vi "Hindbrain Main With Simulator.vi"(11 "NotifierReff":T1) -> ()   [LabVIEW 2013]
doc: "Place to hold all the hindbrain code."
uses:
  Data/TypeDefs/Notifiers.ctl
  Data/TypeDefs/UTM Location.ctl
  Data/TypeDefs/Sail Set Suggestions.ctl
  Data/TypeDefs/Rudder Set Suggestions.ctl
  Data/TypeDefs/OverrideInformation.ctl
  Data/TypeDefs/OverrideMode.ctl
  Data/TypeDefs/MotorSetup.ctl
  Data/TypeDefs/DynamixelSetupInfo.ctl
  Data/TypeDefs/AirmarStatus.ctl
  Data/TypeDefs/HardwareOnline.ctl
  Data/TypeDefs/DynamixelCycleTracker.ctl
  Data/TypeDefs/RC Input Values.ctl
  Classes/Waypoint/Waypoint.lvclass
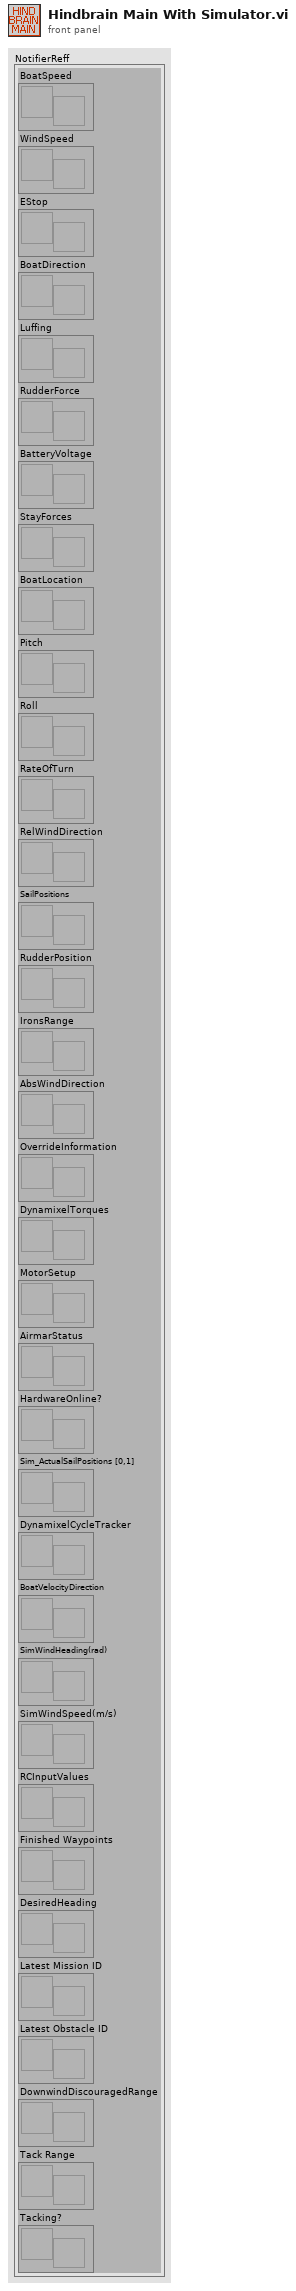
[diagram p1: front panel]
types:
  T1 = typedef "Notifiers.ctl" = cluster{"BoatSpeed":refnum<notifier>, "WindSpeed":refnum<notifier>, "EStop":refnum<notifier>, "BoatDirection":refnum<notifier>, "Luffing":refnum<notifier>, "RudderForce":refnum<notifier>, "BatteryVoltage":refnum<notifier>, "StayForces":refnum<notifier>, "BoatLocation":refnum<notifier>, "Pitch":refnum<notifier>, "Roll":refnum<notifier>, "RateOfTurn":refnum<notifier>, "RelWindDirection":refnum<notifier>, "SailPositions":refnum<notifier>, "RudderPosition":refnum<notifier>, "IronsRange":refnum<notifier>, "AbsWindDirection":refnum<notifier>, "OverrideInformation":refnum<notifier>, "DynamixelTorques":refnum<notifier>, "MotorSetup":refnum<notifier>, "AirmarStatus":refnum<notifier>, "HardwareOnline?":refnum<notifier>, "Sim_ActualSailPositions [0,1]":refnum<notifier>, "DynamixelCycleTracker":refnum<notifier>, "BoatVelocityDirection":refnum<notifier>, "SimWindHeading(rad)":refnum<notifier>, "SimWindSpeed(m/s)":refnum<notifier>, "RCInputValues":refnum<notifier>, "Finished Waypoints":refnum<notifier>, "DesiredHeading":refnum<notifier>, "Latest Mission ID":refnum<notifier>, "Latest Obstacle ID":refnum<notifier>, "DownwindDiscouragedRange":refnum<notifier>, "Tack Range":refnum<notifier>, "Tacking?":refnum<notifier>}
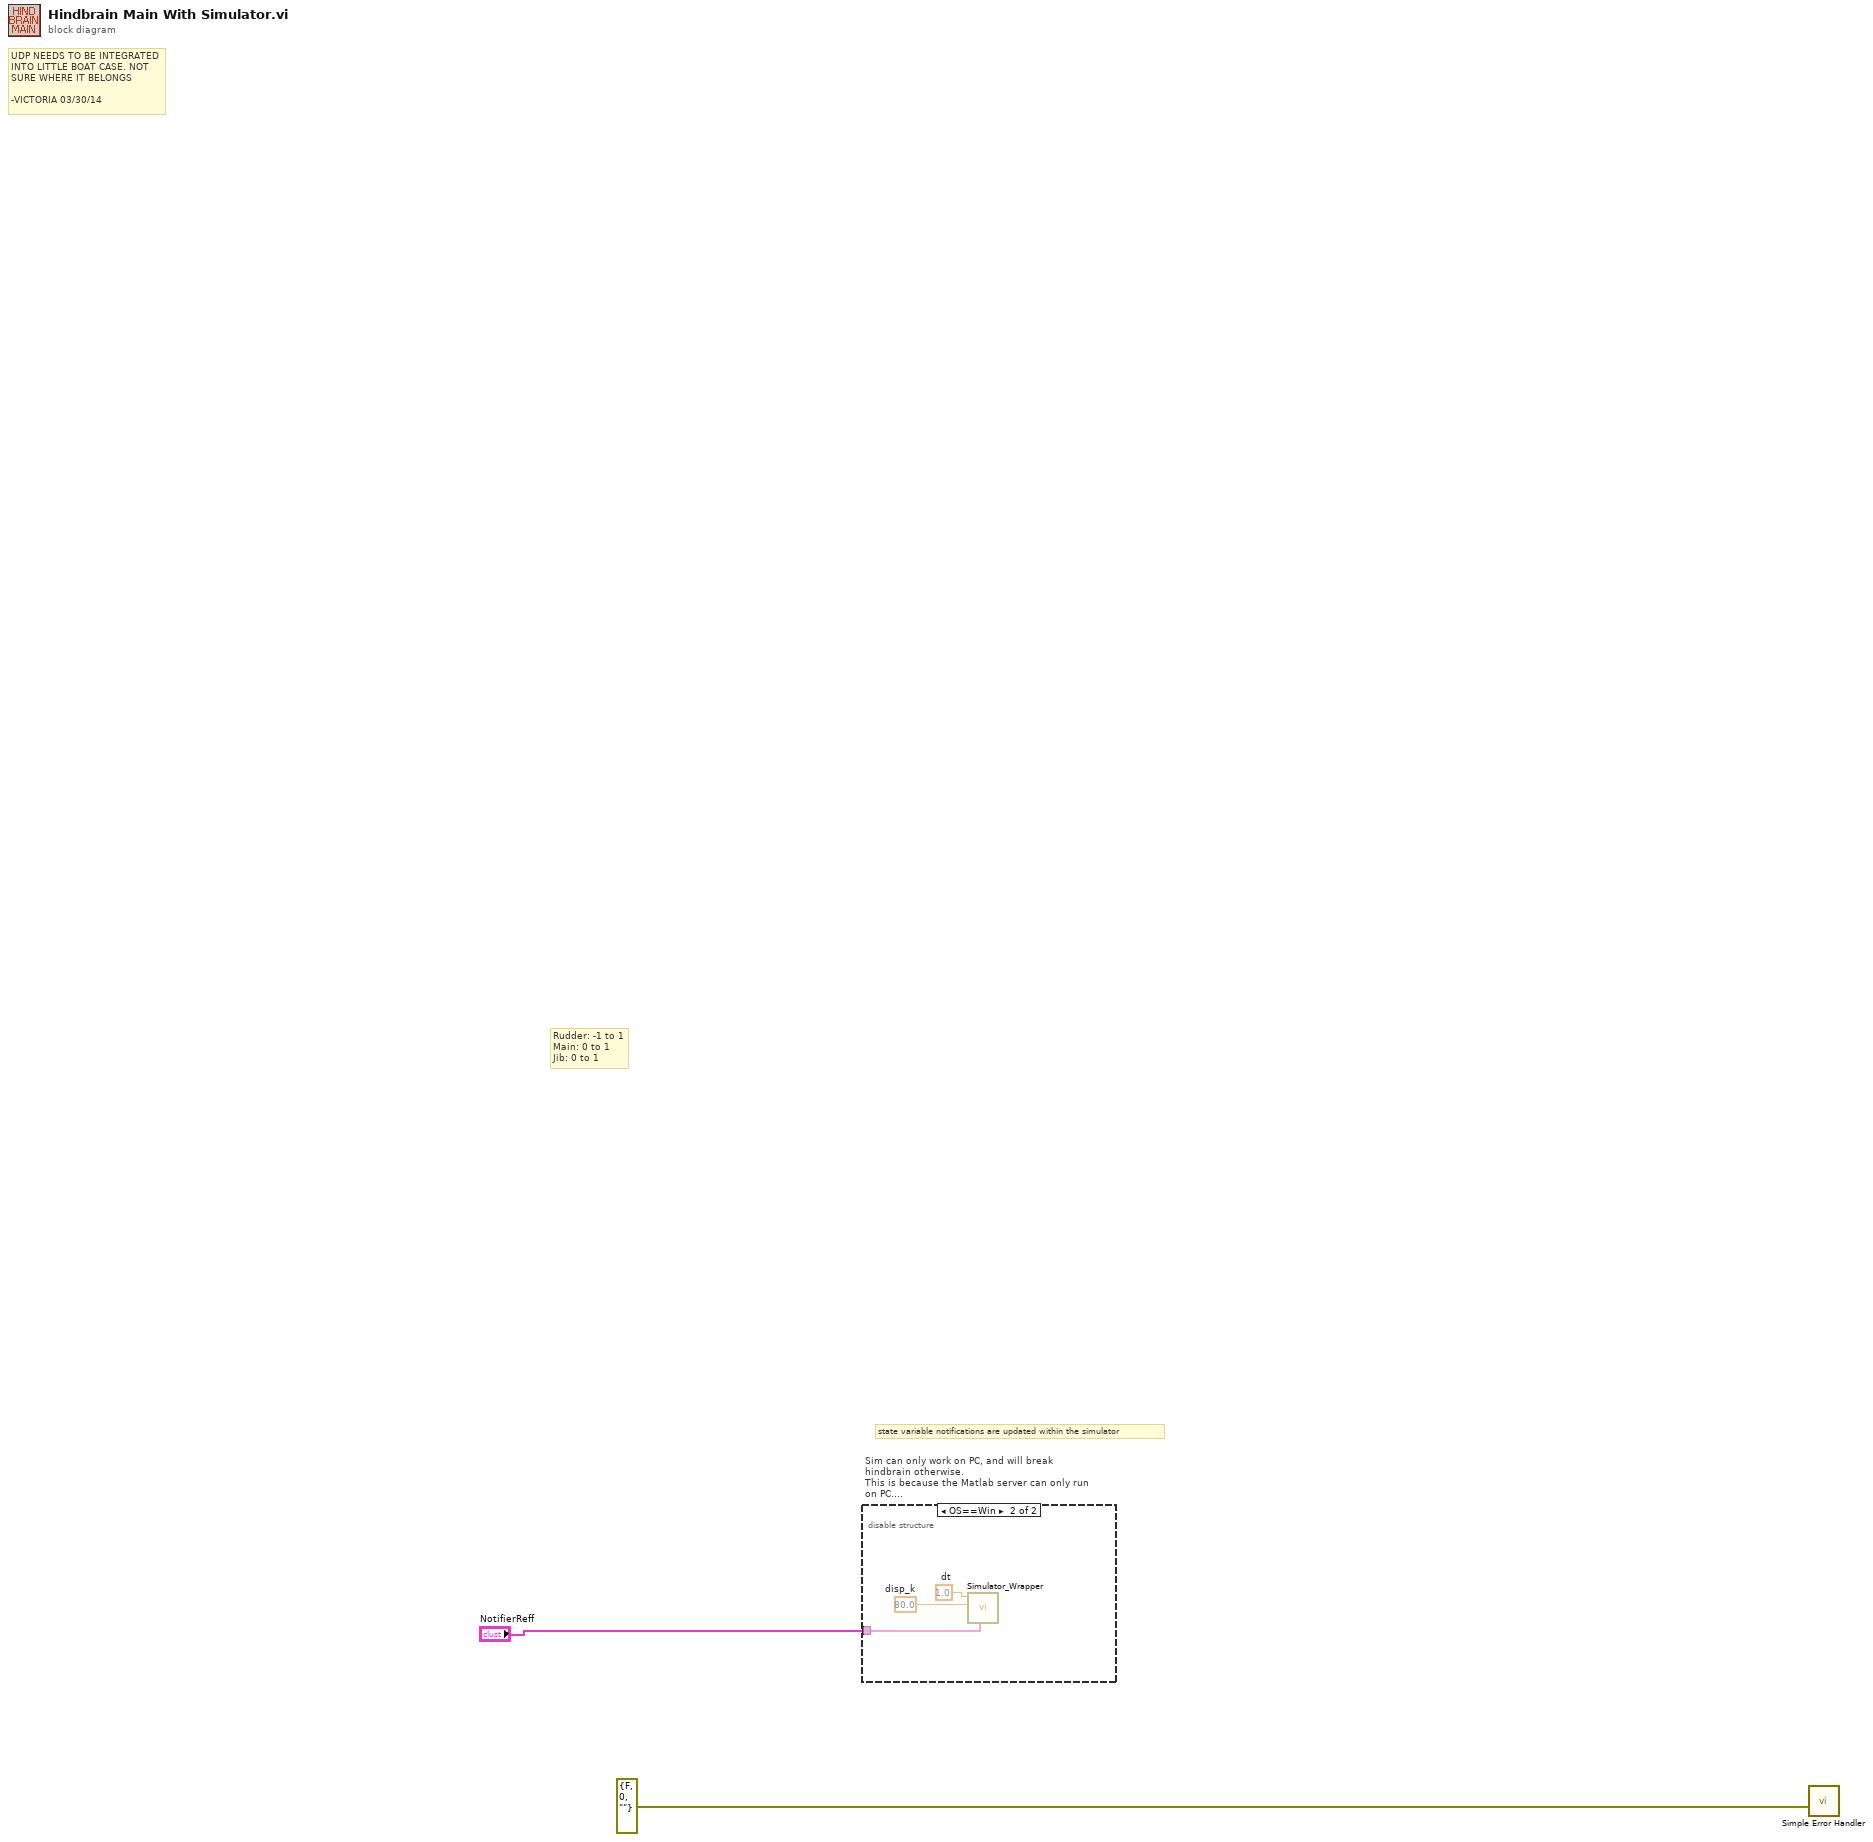
[diagram p0: block diagram]
diagram:
  # "state variable notifications are updated within the simulator"
  # "Rudder: -1 to 1\nMain: 0 to 1 \nJib: 0 to 1"
  # "UDP NEEDS TO BE INTEGRATED\nINTO LITTLE BOAT CASE. NOT \nSURE WHERE IT BELONGS\n\n-VICTORIA 03/30/14"
  n1 = disable-structure "Sim can only work on PC, and will break hindbrain otherwise.\nThis is because the Matlab server can only run on PC.\nTherefore, we have to actually disable (not just case structure)\nthe simulator when not on PC." shown="OS==Win" {
    disable-tunnel: "NotifierReff" -> [_ w4]
    frame condition #0 (active) {
    }
    frame condition #1 {
      w3 = 80.0  # disp_k
      w5 = 1.0  # dt
      n2 = call "Simulator_Wrapper.vi"("NotifierReff"=w4, "disp_k"=w3, "dt"=w5) -> ()  [unwired: 9 in]
    }
  }
  n3 = call <vilib>:"Simple Error Handler.vi"("error in (no error)"=errorcluster {"status"=FALSE, "code"=0, "source"=""} ("error IO")) -> ()  [unwired: 4 in, 5 out]
